vi "读取数据库.vi"(5 "精度(6)":i16=2, 7 "condition":string, 8 "error in (no error)":errorcluster caption="错误输入（无错误）", 9 "database":string="database1.mdb", 10 "显示项":string[](array[string]), 11 "组合框":string(combo)) -> (0 "error out":errorcluster caption="错误输出", 1 "columns":string[](array[string]), 2 "data":variant[][](array[variant]), 3 "表格":string[][](table))   [LabVIEW 2016]
uses:
  <vilib>/Utility/sysdir.llb/System Directory Type.ctl
  <vilib>/addons/database/Connection.llb/DB Tools Open Connec (String).vi
  <vilib>/addons/database/_DB Variant To Data/Database Variant To Data.xnode
  <vilib>/addons/database/NI_Database_API.lvlib
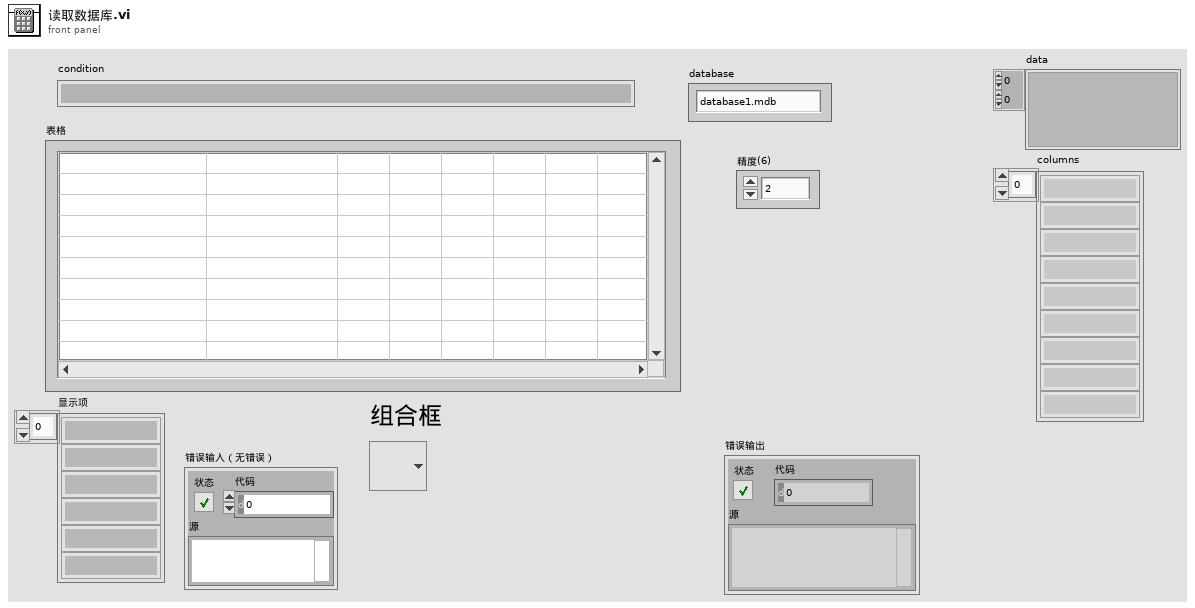
[diagram p1: front panel]
types:
  T1 = typedef "System Directory Type.ctl" = i32
  T2 = typedef "NI_Database_API.lvlib/Conn ObjectReference.ctl" = refnum<k1>
  T3 = typedef "NI_Database_API.lvlib/DB Tools DataTypes.ctl" = enum16{"String", "Long (I32)", "Single (SGL)", "Double (DBL)", "Date/Time", "Binary"}
  T4 = cluster{"name":string, "database data type":T3, "defined size":i32}[]
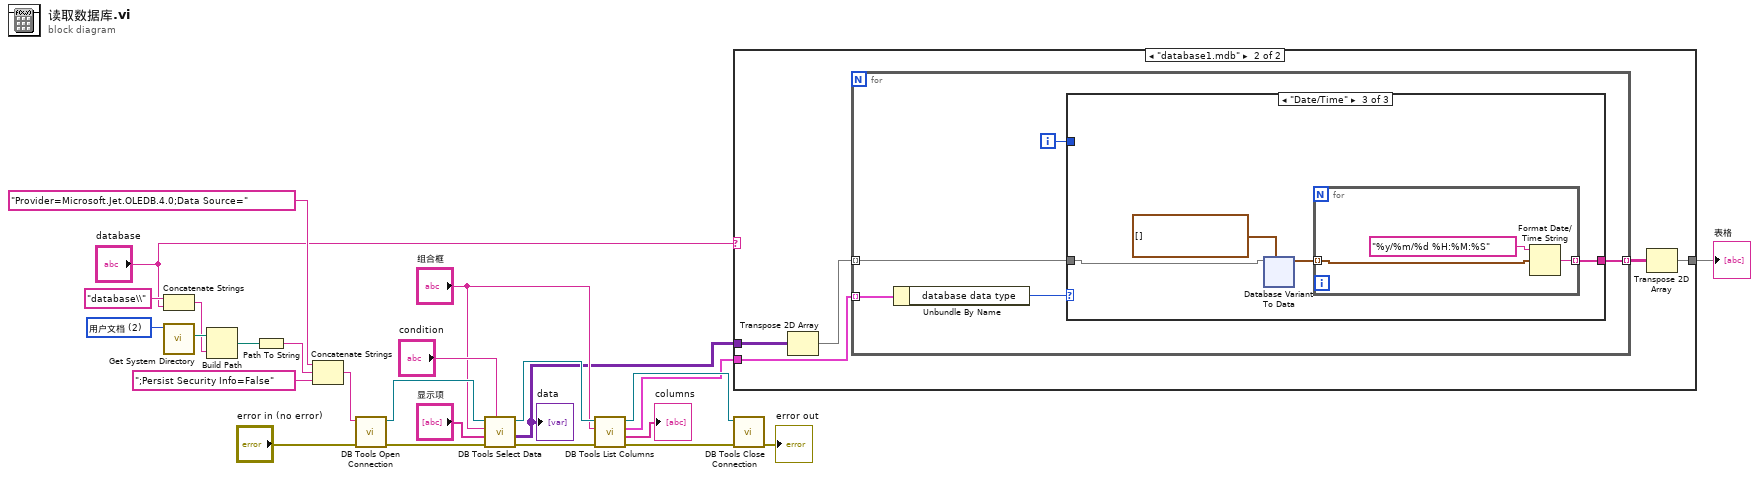
[diagram p0: block diagram]
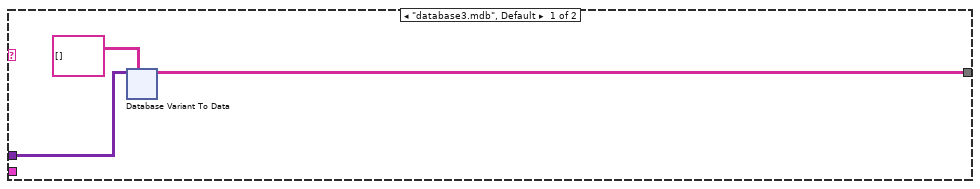
[diagram p2: hidden frame]
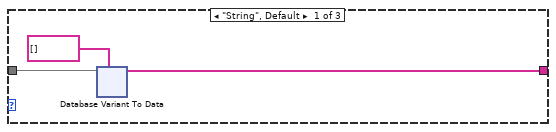
[diagram p3: hidden frame]
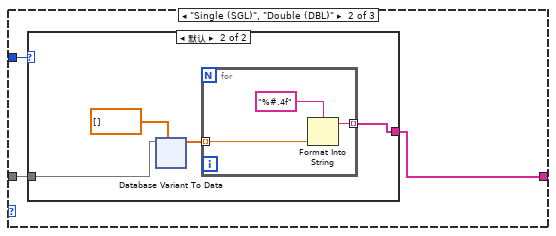
[diagram p4: hidden frame]
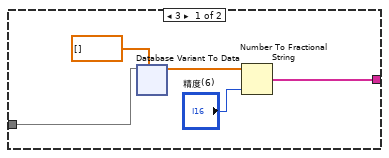
[diagram p5: hidden frame]
diagram:
  w10 = T1 2 items=["用户目录"=0, "用户桌面"=1, "用户文档"=2, "用户应用程序数据"=3, "用户设置"=4, "用户临时目录"=5, "公共文档"=6, "公共应用程序数据"=7, "公共设置"=8, "公共缓存"=13, "系统核心库"=9, "系统安装库"=10, "应用程序文件"=11, "启动盘根目录"=12] ("system directory type")
  n1 = Concatenate Strings("database\\" ("名称或相对路径"), "database") -> (w6:string)
  n2 = call <vilib>:"Get System Directory.vi"("system directory type"=w10) -> ("system directory"=w9:path)  [unwired: 10 in]
  n3 = Build Path(base path=w9, name or relative path=w6) -> (appended path=w11:path)
  n4 = Path To String(path=w11) -> (string=w12:string)
  n5 = Concatenate Strings("Provider=Microsoft.Jet.OLEDB.4.0;Data Source=", w12, ";Persist Security Info=False") -> (w8:string)
  n6 = call-poly <vilib>:"DB Tools Open Connection.vi"("error in (no error)"="error in (no error)", "connection information"=w8) -> ("error out"=w24:errorcluster, "connection reference"=w25:T2)  [unwired: 6 in]
  n7 = call <vilib>:"DB Tools Select Data.vi"("condition"="condition", "error in (no error)"=w24, "columns"="显示项", "table"="组合框", "connection reference"=w25) -> ("error out"=w23:errorcluster, "data"=w4:variant[][], "connection reference out"=w20:T2)  [unwired: 1 in]
  "data" <- w4
  n8 = call <vilib>:"DB Tools List Columns.vi"("error in (no error)"=w23, "table"="组合框", "connection reference"=w20) -> ("error out"=w15:errorcluster, "columns"=→"columns":string[], "column information"=w3:T4, "connection reference out"=w16:T2)  [unwired: 1 in]
  n9 = case shown="\"database1.mdb\"" "database" {
    tunnel: w4 -> [w27 w77]
    tunnel: w3 -> [_ w75]
    tunnel: [w26 w73] -> w2
    frame "database3.mdb", Default {
      n10 = xnode "Database Variant To Data"("database variant"=w27, "type"=string[][] []) -> ("data"=w26:string[][])  [unwired: 1 in, 1 out]
    }
    frame "database1.mdb" {
      n11 = Transpose 2D Array(2D array=w77) -> (transposed array=w76:variant[][])
      n12 = for {
        tunnel: w76 -> [w80] mode=indexing
        tunnel: w75 -> [w82] mode=indexing
        tunnel: [w79] -> w74 mode=indexing
        i -> [w78]
        n13 = Unbundle By Name(w82) -> ("database data type"=w81:T3)
        n14 = case shown="\"Date/Time\"" w81 {
          tunnel: w80 -> [w84 w126 w217]
          tunnel: [w83 w125 w215] -> w79
          tunnel: w78 -> [_ w124 _]
          frame "String", Default {
            n15 = xnode "Database Variant To Data"("database variant"=w84, "type"=string[] []) -> ("data"=w83:string[])  [unwired: 1 in, 1 out]
          }
          frame "Single (SGL)", "Double (DBL)" {
            n16 = case shown="默认" w124 {
              tunnel: w126 -> [w131 w172]
              tunnel: [w127 w170] -> w125
              frame 3 {
                n17 = xnode "Database Variant To Data"("database variant"=w131, "type"=dbl[] []) -> ("data"=w129:dbl[])  [unwired: 1 in, 1 out]
                n18 = Number To Fractional String(number=w129, precision (6)="精度(6)") -> (F-format string=w127:string[])  [unwired: 2 in]
              }
              frame Default {
                n19 = xnode "Database Variant To Data"("database variant"=w172, "type"=dbl[] []) -> ("data"=w171:dbl[])  [unwired: 1 in, 1 out]
                n20 = for {
                  tunnel: w171 -> [w176] mode=indexing
                  tunnel: [w174] -> w170 mode=indexing
                  n21 = Format Into String(format string="%#.4f" ("格式字符串"), w176) -> (resulting string=w174:string)  [unwired: 2 in, 1 out]
                }
              }
            }
          }
          frame "Date/Time" {
            n22 = xnode "Database Variant To Data"("database variant"=w217, "type"=timestamp[] []) -> ("data"=w216:timestamp[])  [unwired: 1 in, 1 out]
            n23 = for {
              tunnel: w216 -> [w220] mode=indexing
              tunnel: [w219] -> w215 mode=indexing
              n24 = Format Date/Time String(time format string (%c)="%y/%m/%d %H:%M:%S" ("时间格式字符串(%c)"), seconds (now)=w220) -> (date/time string=w219:string)  [unwired: 1 in]
            }
          }
        }
      }
      n25 = Transpose 2D Array(2D array=w74) -> (transposed array=w73:string[][])
    }
  }
  "表格" <- w2
  n26 = call <vilib>:"DB Tools Close Connection.vi"("error in (no error)"=w15, "connection reference"=w16) -> ("error out"=→"error out":errorcluster)  [unwired: 5 in]
